vi "PolarizationSimulation.vi"() -> ()   [LabVIEW 2018]
uses:
  Sub-VI's/Adam_data.ctl
  <vilib>/Utility/xml.llb/Read From XML File(string).vi
  <vilib>/Utility/xml.llb/Write to XML File(string).vi
  <vilib>/Analysis/NI_AALBase.lvlib
panel:
  in  "Regularization":T1
  in  "Batch Size":i16
  out "NN Loss":dbl(graph)
  in  "Loss Function":enum16{"MSE", "MAE"}(ring)
  in  "Parameters File Path":path
  out "NN Error":dbl
  in  "Training?":bool
  out "NN Output":dbl
  in  "Speed\nMultiplier":dbl=1.0
  out "Rho_-":cluster{dbl[], "Array 3":dbl[]}(graph)
  out "Rho_0":cluster{dbl[], "Array out":dbl[]}(graph)
  in  "AFP On":bool
  in  "AFP Efficiency":dbl=0.9 min=0.0 max=1.0 step=0.01
  in  "AFP Control":cluster{i32, i32}(slide)={200, 230} scale=0.0..500.0
  out "lower R-value AFP":dbl
  out "upper R-value AFP":dbl
  in  "STOP":bool
  in  "Microwave Power":dbl=1.0
  in  "Lower Fit\nParameter":dbl=-3.6
  in  "Upper Fit\nParameter":dbl=3.6
  in  "Std Dev Noise":dbl step=0.0001
  out "lower R-value":dbl
  out "upper R-value":dbl
  in  "RF Control":cluster{i32, i32}(slide)={200, 230} scale=0.0..500.0
  out "p":dbl format="%_4g"
  out "r":dbl
  in  "Saturation\nPolarization":dbl=0.8 min=0.0 max=0.99 step=0.01
  out "Reimann \nsum of Q":dbl format="%_4g"
  out "Corrected Data (Q)":cluster{dbl[], dbl[]}(graph)
  out "Rho_+":cluster{dbl[], "Array out":dbl[]}(graph)
  in  "Select Target Type":u16(ring)=2 items=["Test Case", "Deuteron"]
  in  "Reset":bool
  out "Total Polarization (P)":cluster{dbl, dbl}(graph)
  in  "Spin Manipulation\nPower Factor":dbl=0.005
  in  "Decay Spin\nManipulation":bool
  out "Reimann\nsum of P":dbl format="%_4g"
  out "Corrected Data (P)":cluster{dbl[], dbl[]}[](graph)
  out "Signal and Fit (P)":cluster{dbl[], "Best Polynomial Fit":dbl[]}[](graph)
  in  "Positive\nPolarization":bool
  in  "Microwave on":bool
  # "Neural Network"
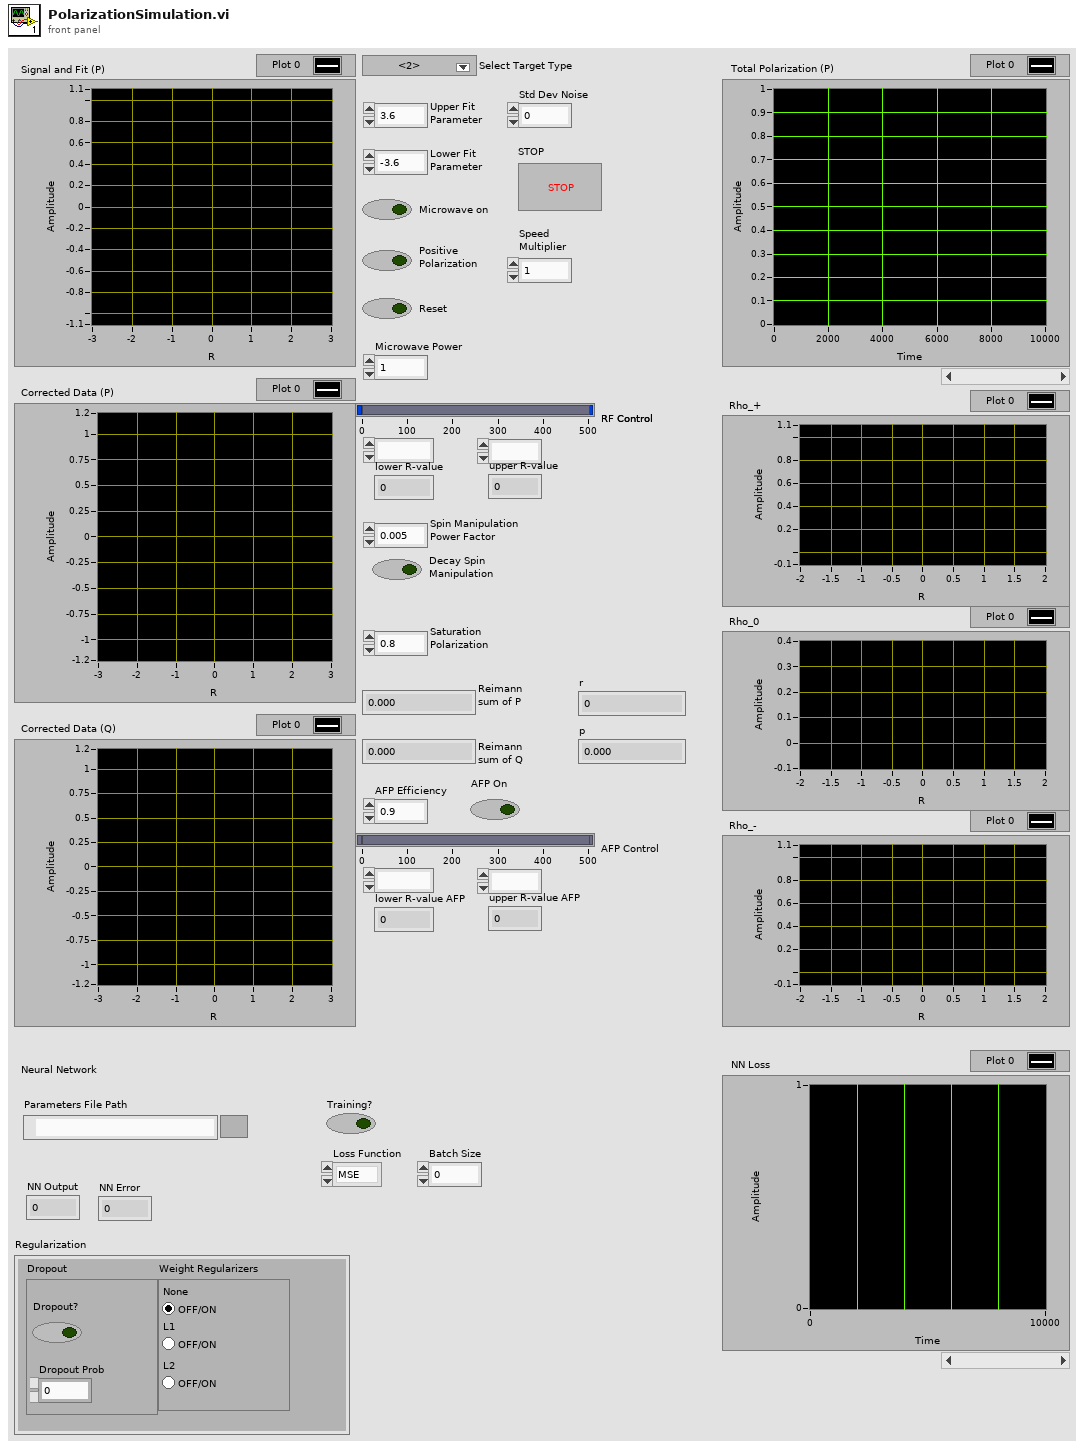
[diagram p1: front panel]
types:
  T1 = cluster{"Dropout":cluster{"Dropout?":bool, "Dropout Prob":dbl}, "Weight Regularizers":enum32{"None", "L1", "L2"}}
  T2 = typedef "Adam_data.ctl" = cluster{"Mw Moments":cluster{"3 ":dbl[], "2":dbl[][], "1":dbl[][]}, "Vw Moments":cluster{"3":dbl[], "2":dbl[][], "1":dbl[][]}, "Mb Moments":cluster{"3":dbl, "2":dbl[], "1":dbl[]}, "Vb Moments":cluster{"3":dbl, "2":dbl[], "1":dbl[]}}
  T3 = cluster{cluster{dbl[][], dbl[]}, cluster{dbl[][], dbl[]}, cluster{dbl[], dbl}}
  T4 = cluster{cluster{"Updated Weights":dbl[][], "Updated Biases":dbl[]}, cluster{"Updated Weights":dbl[][], "Updated Biases":dbl[]}, cluster{"Updated Weights":dbl[], "Updated Biases":dbl}}
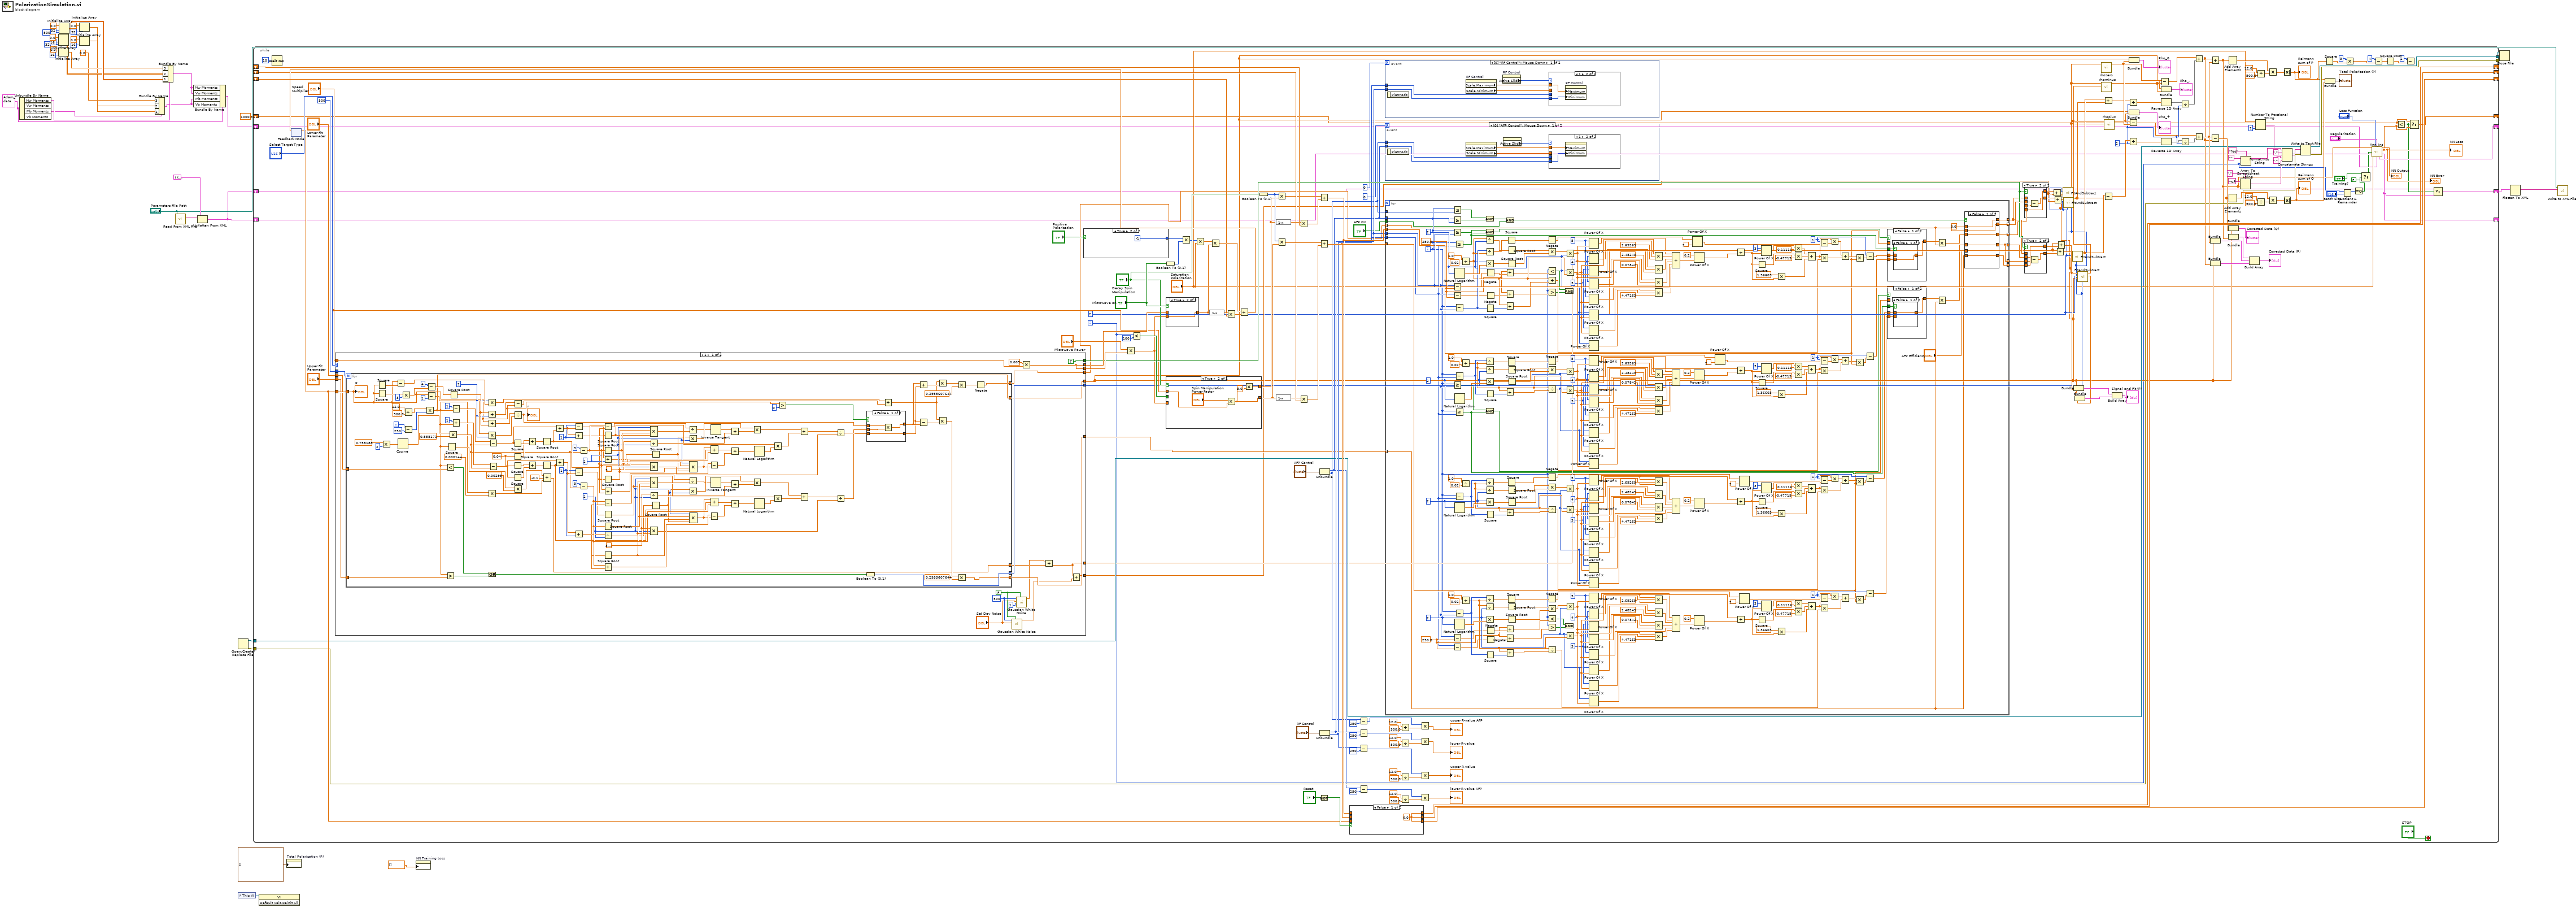
[diagram p0: block diagram]
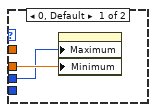
[diagram p2: hidden frame]
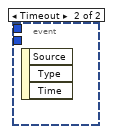
[diagram p3: hidden frame]
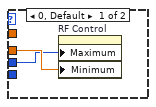
[diagram p4: hidden frame]
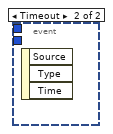
[diagram p5: hidden frame]
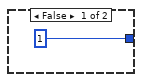
[diagram p6: hidden frame]
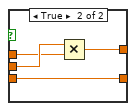
[diagram p7: hidden frame]
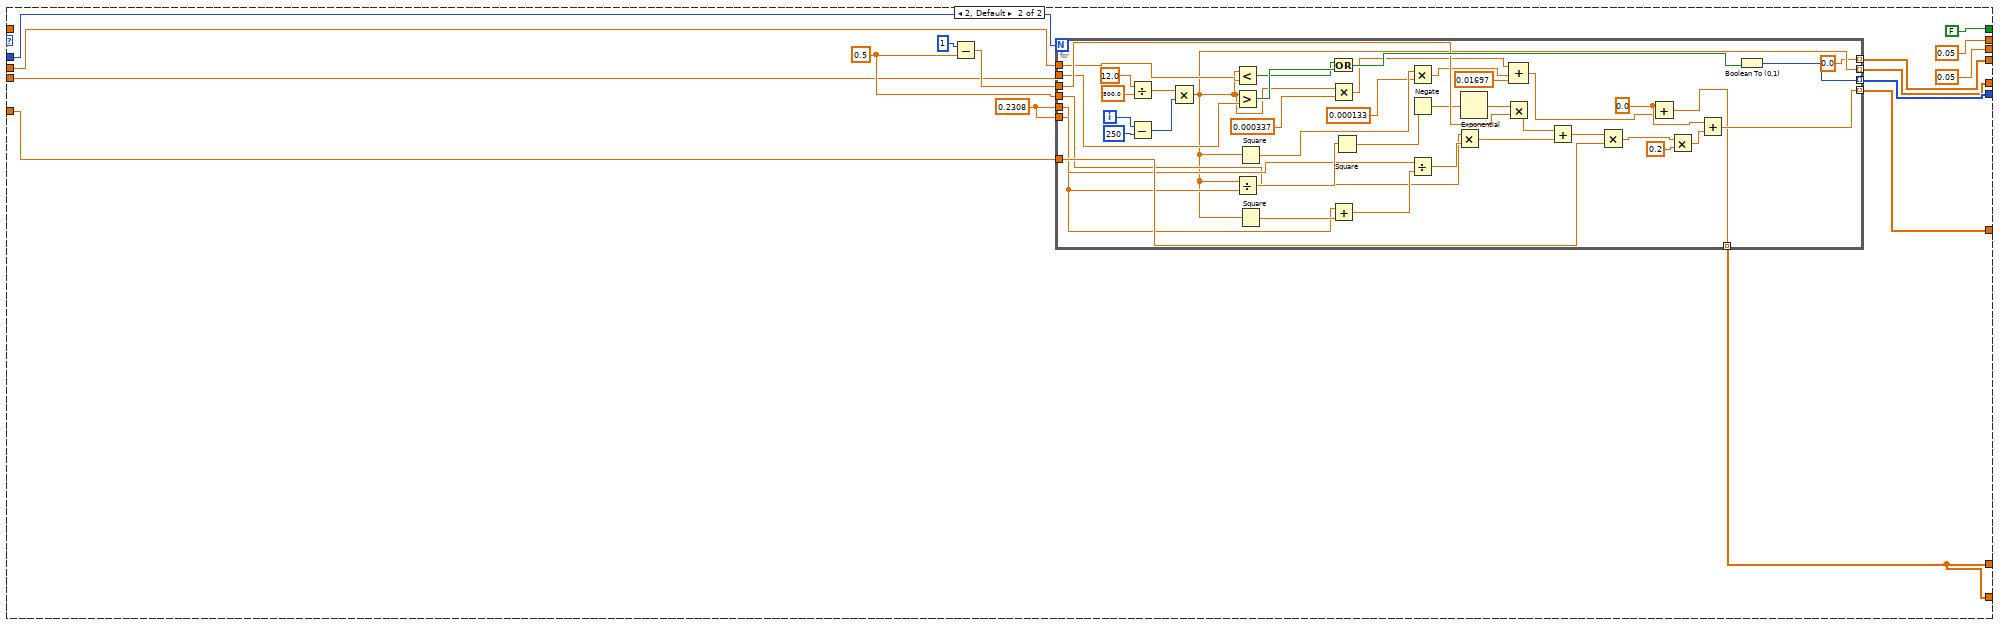
[diagram p8: hidden frame]
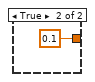
[diagram p10: hidden frame]
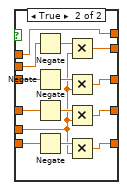
[diagram p15: hidden frame]
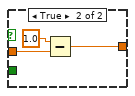
[diagram p17: hidden frame]
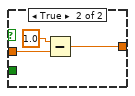
[diagram p19: hidden frame]
diagram:
  w7 = T2 {"Mw Moments"={"3 "=[], "2"=[], "1"=[]}, "Vw Moments"={"3"=[], "2"=[], "1"=[]}, "Mb Moments"={"3"=0.0, "2"=[], "1"=[]}, "Vb Moments"={"3"=0.0, "2"=[], "1"=[]}} ("Adam Data In")
  n1 = Unbundle By Name(w7) -> ("Mw Moments"=w9:cluster{"3 ":dbl[], "2":dbl[][], "1":dbl[][]}, "Mb Moments"=w8:cluster{"3":dbl, "2":dbl[], "1":dbl[]})  [unwired: 2 out]
  n2 = Initialize Array(0.0 ("element"), 16 ("dimension size"), 32 ("dimension size")) -> (w14:dbl[][])
  n3 = Initialize Array(0.0 ("element"), 16 ("dimension size")) -> (w13:dbl[])
  n4 = Initialize Array(0.0 ("element"), 32 ("dimension size"), 500 ("dimension size")) -> (w15:dbl[][])
  n5 = Initialize Array(0.0 ("element"), 16 ("dimension size")) -> (w11:dbl[])
  n6 = Initialize Array(0.0 ("element"), 32 ("dimension size")) -> (w12:dbl[])
  n7 = Bundle By Name(cluster=w8, "3"=0.0 ("element"), "2"=w11, "1"=w12) -> (w5:cluster{"3":dbl, "2":dbl[], "1":dbl[]})
  n8 = Bundle By Name(cluster=w9, "3"=w13, "2"=w14, "1"=w15) -> (w6:cluster{"3 ":dbl[], "2":dbl[][], "1":dbl[][]})
  n9 = call-poly <vilib>:"Read From XML File.vi"("XML File Path"="Parameters File Path") -> ("XML Elements"=w32:string)  [unwired: 8 in, 2 out]
  n10 = Bundle By Name(cluster=w7, "Mw Moments"=w6, "Vw Moments"=w6, "Mb Moments"=w5, "Vb Moments"=w5) -> (w4:T2)
  n11 = Unflatten From XML(xml string=w32, type=T3 {{[], []}, {[], []}, {[], 0.0}}) -> (value=w3:T3)  [unwired: 1 in, 1 out]
  n12 = Open/Create/Replace File() -> (refnum out=w36:refnum<file>, error out=w35:errorcluster)  [unwired: 6 in, 1 out]
  n13 = control-ref of="This VI"() -> (w38:refnum<vi>)
  n14 = while {
    shift-right: [w215] -> _
    shift-left: _ -> [w222]
    shift-right: [w214] -> _
    shift-left: _ -> [w197]
    shift-right: [w192] -> _
    shift-left: _ -> [w191]
    tunnel: w36 -> [w124]
    tunnel: w35 -> [w123]
    tunnel: [w122] -> w34
    tunnel: [w121] -> w33
    shift-right: [w42] -> _
    shift-left: w3 -> [w58]
    shift-right: [w55] -> _
    shift-left: w4 -> [w54]
    shift-right: [w46] -> _
    shift-left: 1000.0 ("Error") -> [w45]
    shift-right: [w41] -> w2
    shift-left: w3 -> [w40]
    i -> [w53]
    stop <- "STOP" stop-if-true
    w174 = 2
    w67 = 2
    n15 = Wait (ms)(milliseconds to wait=10) -> ()  [unwired: 1 out]
    n16 = feedback #1() -> (w201:dbl)  [unwired: 1 in]
    n17 = case shown="1" "Select Target Type" {
      tunnel: [w257 0.05 ("Growth Constant")] -> w206
      tunnel: [w257 0.05 ("Decay Constant")] -> w205
      tunnel: 500 -> [w266 w424]
      tunnel: w201 -> [w269 w423]
      tunnel: "Upper Fit\nParameter" -> [w267 w421]
      tunnel: "Lower Fit\nParameter" -> [w268 w422]
      tunnel: [w264 w419] -> w66
      tunnel: [w254 w418] -> w81
      tunnel: [w265 w420] -> w65
      tunnel: [TRUE FALSE] -> w185
      tunnel: [w255 w414] -> w80
      tunnel: "Speed\nMultiplier" -> [w256 _]
      tunnel: [w250 w413] -> w79
      tunnel: [w252 w413] -> w78
      frame 1 {
        w259 = FALSE
        w261 = 500
        n18 = for {
          N: w266 -> [_]
          tunnel: [w300] -> w264 mode=indexing
          tunnel: [w389] -> w265 mode=indexing
          tunnel: w267 -> [w388]
          tunnel: w268 -> [w387]
          tunnel: [w272] -> w254 mode=indexing
          tunnel: w269 -> [w273]
          tunnel: [w271] -> w255 mode=indexing
          tunnel: [w270] -> w253 mode=indexing
          i -> [w365]
          w287 = 2
          w326 = 1
          w330 = 3.141592653589793
          w324 = 2
          w309 = 0.04
          w362 = 1
          w367 = 3.141592653589793
          w360 = 2
          n19 = Square(x=w273) -> (x^2=w290:dbl)
          n20 = Square(x=w273) -> (x^2=w316:dbl)
          n21 = Multiply(x=0.758188, y=2) -> (x*y=w304:dbl)
          n22 = Subtract(x=w273, y=w290) -> (x-y=w289:dbl)
          n23 = Cosine(x=w304) -> (cos(x)=w307:dbl)
          n24 = Multiply(x=w316, y=3) -> (x*y=w315:dbl)
          n25 = Divide(x=12.0, y=500.0) -> (x/y=w403:dbl)
          n26 = Subtract(x=w365, y=250) -> (x-y=w402:i32)
          n27 = Multiply(x=w403, y=w402) -> (x*y=w300:dbl)
          n28 = Subtract(x=4, y=w315) -> (x-y=w313:dbl)
          n29 = Subtract(x=w273, y=1) -> (x-y=w311:dbl)
          n30 = Less?(x=w300, y=w387) -> (x < y?=w392:bool)
          n31 = Greater?(x=w300, y=w388) -> (0:w391:bool)
          n32 = Square(x=w300) -> (x^2=w302:dbl)
          n33 = Multiply(x=w307, y=0.558171) -> (x*y=w308:dbl)
          n34 = Square Root(x=w313) -> (sqrt(x)=w288:dbl)
          n35 = Subtract(x=1, y=w300) -> (x-y=w397:dbl)
          n36 = Add(x=1, y=w300) -> (x+y=w354:dbl)
          n37 = Multiply(x=w287, y=w289) -> (x*y=w285:dbl)
          n38 = Add(x=w288, y=w287) -> (x+y=w286:dbl)
          n39 = Add(x=w273, y=w288) -> (x+y=w312:dbl)
          n40 = Multiply(x=w311, y=w287) -> (x*y=w295:dbl)
          n41 = Multiply(x=w300, y=0.000144) -> (x*y=w297:dbl)
          n42 = Or(x=w392, y=w391) -> (x .or. y?=w390:bool)
          n43 = Subtract(x=w397, y=w308) -> (x-y=w393:dbl)
          n44 = Subtract(x=w354, y=w308) -> (x-y=w350:dbl)
          n45 = Square(x=w393) -> (x^2=w396:dbl)
          n46 = Square(x=w309) -> (x^2=w395:dbl)
          n47 = Square(x=w309) -> (x^2=w352:dbl)
          n48 = Square(x=w350) -> (x^2=w353:dbl)
          n49 = Subtract(x=w286, y=w273) -> (x-y=w284:dbl)
          n50 = Divide(x=w312, y=w295) -> (x/y=w291:dbl)
          "r" <- w291
          n51 = Multiply(x=w302, y=0.00295) -> (x*y=w301:dbl)
          n52 = Add(x=w395, y=w396) -> (x+y=w394:dbl)
          n53 = Add(x=w352, y=w353) -> (x+y=w351:dbl)
          n54 = Square Root(x=w394) -> (sqrt(x)=w357:dbl)
          n55 = Square Root(x=w351) -> (sqrt(x)=w321:dbl)
          n56 = Compound Arithmetic op=ADD(w301, -0.1, w297) -> (w270:dbl)
          n57 = Divide(x=w393, y=w357) -> (x/y=w363:dbl)
          n58 = Divide(x=w350, y=w321) -> (x/y=w327:dbl)
          n59 = Subtract(x=w362, y=w363) -> (x-y=w318:dbl)
          n60 = Add(x=w363, y=w362) -> (x+y=w361:dbl)
          n61 = Subtract(x=w326, y=w327) -> (x-y=w319:dbl)
          n62 = Add(x=w327, y=w326) -> (x+y=w325:dbl)
          n63 = Subtract(x=3, y=w308) -> (x-y=w373:dbl)
          n64 = Subtract(x=3, y=w308) -> (x-y=w336:dbl)
          n65 = Subtract(x=w373, y=w357) -> (x-y=w382:dbl)
          n66 = Square Root(x=w318) -> (sqrt(x)=w364:dbl)
          n67 = Square Root(x=w373) -> (sqrt(x)=w376:dbl)
          n68 = Divide(x=w361, y=w360) -> (x/y=w359:dbl)
          n69 = Square Root(x=w357) -> (sqrt(x)=w366:dbl)
          n70 = Add(x=w373, y=w357) -> (x+y=w372:dbl)
          n71 = Subtract(x=w336, y=w321) -> (x-y=w345:dbl)
          n72 = Square Root(x=w319) -> (sqrt(x)=w328:dbl)
          n73 = Square Root(x=w336) -> (sqrt(x)=w339:dbl)
          n74 = Divide(x=w325, y=w324) -> (x/y=w323:dbl)
          n75 = Square Root(x=w321) -> (sqrt(x)=w329:dbl)
          n76 = Add(x=w336, y=w321) -> (x+y=w335:dbl)
          n77 = Divide(x=w367, y=w360) -> (x/y=w384:dbl)
          n78 = Divide(x=w330, y=w324) -> (x/y=w347:dbl)
          n79 = Compound Arithmetic op=MULTIPLY(w360, w366, w376, w364) -> (w381:dbl)
          n80 = Compound Arithmetic op=MULTIPLY(w367, w360, w366) -> (w368:dbl)
          n81 = Compound Arithmetic op=MULTIPLY(w324, w329, w339, w328) -> (w344:dbl)
          n82 = Compound Arithmetic op=MULTIPLY(w330, w324, w329) -> (w331:dbl)
          n83 = Square Root(x=w359) -> (sqrt(x)=w358:dbl)
          n84 = Square Root(x=w323) -> (sqrt(x)=w322:dbl)
          n85 = Divide(x=w382, y=w381) -> (x/y=w380:dbl)
          n86 = Multiply(x=w358, y=w360) -> (x*y=w386:dbl)
          n87 = Divide(x=w345, y=w344) -> (x/y=w343:dbl)
          n88 = Multiply(x=w322, y=w324) -> (x*y=w349:dbl)
          n89 = Compound Arithmetic op=MULTIPLY(w360, w376, w366, w358) -> (w371:dbl)
          n90 = Compound Arithmetic op=MULTIPLY(w324, w339, w329, w322) -> (w334:dbl)
          n91 = Subtract(x=w372, y=w371) -> (x-y=w370:dbl)
          n92 = Subtract(x=w335, y=w334) -> (x-y=w333:dbl)
          n93 = Inverse Tangent(1:w380) -> (0:w385:dbl)
          n94 = Compound Arithmetic op=ADD(w371, w357, w373) -> (w375:dbl)
          n95 = Inverse Tangent(1:w343) -> (0:w348:dbl)
          n96 = Compound Arithmetic op=ADD(w334, w321, w336) -> (w338:dbl)
          n97 = Add(x=w385, y=w384) -> (x+y=w383:dbl)
          n98 = Divide(x=w375, y=w370) -> (x/y=w374:dbl)
          n99 = Add(x=w348, y=w347) -> (x+y=w346:dbl)
          n100 = Divide(x=w338, y=w333) -> (x/y=w337:dbl)
          n101 = Multiply(x=w386, y=w383) -> (x*y=w379:dbl)
          n102 = Multiply(x=w349, y=w346) -> (x*y=w342:dbl)
          n103 = Natural Logarithm(1:w374) -> (0:w377:dbl)
          n104 = Natural Logarithm(1:w337) -> (0:w340:dbl)
          n105 = Multiply(x=w364, y=w377) -> (x*y=w378:dbl)
          n106 = Multiply(x=w328, y=w340) -> (x*y=w341:dbl)
          n107 = Greater?(x=w273, y=0) -> (0:w275:bool)
          n108 = Add(x=w379, y=w378) -> (x+y=w369:dbl)
          n109 = Add(x=w342, y=w341) -> (x+y=w332:dbl)
          n110 = Divide(x=w369, y=w368) -> (x/y=w310:dbl)
          n111 = Divide(x=w332, y=w331) -> (x/y=w277:dbl)
          n112 = Boolean To (0,1)(Boolean=w390) -> (0, 1=w389:i16)
          n113 = case shown="False" w275 {
            tunnel: w310 -> [w407 w412]
            tunnel: [w405 w411] -> w293
            tunnel: w291 -> [w408 w410]
            tunnel: w277 -> [w406 w409]
            tunnel: [w406 w409] -> w276
            frame False {
              n114 = Multiply(x=w408, y=w407) -> (x*y=w405:dbl)
            }
            frame True {
              n115 = Multiply(x=w412, y=w410) -> (x*y=w411:dbl)
            }
          }
          n116 = Divide(x=w285, y=w284) -> (x/y=w283:dbl)
          n117 = Add(x=w293, y=w276) -> (x+y=w294:dbl)
          n118 = Subtract(x=w276, y=w293) -> (x-y=w320:dbl)
          n119 = Multiply(x=w283, y=w294) -> (x*y=w282:dbl)
          n120 = Multiply(x=w283, y=w320) -> (x*y=w281:dbl)
          n121 = Multiply(x=w282, y=0.2955607644) -> (x*y=w280:dbl)
          n122 = Multiply(x=w281, y=0.2955607644) -> (x*y=w272:dbl)
          n123 = Negate(x=w280) -> (-x=w271:dbl)
          "p" <- w273
        }
        n124 = call <vilib>:"Gaussian White Noise.vi"("initialize?"=w259, "standard deviation"="Std Dev Noise", "samples"=w261) -> ("Gaussian noise pattern"=w251:dbl[])  [unwired: 7 in, 1 out]
        n125 = call <vilib>:"Gaussian White Noise.vi"("initialize?"=w259, "seed"=1, "standard deviation"="Std Dev Noise", "samples"=w261) -> ("Gaussian noise pattern"=w249:dbl[])  [unwired: 6 in, 1 out]
        n126 = Multiply(x=0.005, y=w256) -> (x*y=w257:dbl)
        n127 = Add(x=w249, y=w253) -> (x+y=w250:dbl[])
        n128 = Add(x=w250, y=w251) -> (x+y=w252:dbl[])
      }
      frame 2, Default {
        w425 = 0.2308
        w426 = 0.5
        n129 = Subtract(x=1, y=w426) -> (x-y=w428:dbl)
        n130 = for {
          N: w424 -> [_]
          tunnel: w423 -> [w468]
          tunnel: [w434] -> w419 mode=indexing
          tunnel: [w452] -> w418 mode=indexing
          tunnel: [w466] -> w420 mode=indexing
          tunnel: w428 -> [w462]
          tunnel: w425 -> [w460]
          tunnel: w425 -> [w441]
          tunnel: w426 -> [w454]
          tunnel: w421 -> [w449]
          tunnel: w422 -> [w448]
          tunnel: [0.0] -> w414 mode=indexing
          tunnel: [w429] -> w413 mode=indexing
          i -> [w442]
          w453 = 0.0
          n131 = Divide(x=12.0, y=500.0) -> (x/y=w443:dbl)
          n132 = Subtract(x=w442, y=250) -> (x-y=w447:i32)
          n133 = Multiply(x=w443, y=w447) -> (x*y=w434:dbl)
          n134 = Less?(x=w434, y=w448) -> (x < y?=w463:bool)
          n135 = Greater?(x=w434, y=w449) -> (0:w464:bool)
          n136 = Divide(x=w434, y=w441) -> (x/y=w469:dbl)
          n137 = Square(x=w434) -> (x^2=w437:dbl)
          n138 = Square(x=w434) -> (x^2=w459:dbl)
          n139 = Or(x=w463, y=w464) -> (x .or. y?=w465:bool)
          n140 = Multiply(x=w434, y=0.000337) -> (x*y=w436:dbl)
          n141 = Add(x=w441, y=w459) -> (x+y=w461:dbl)
          n142 = Square(x=w469) -> (x^2=w470:dbl)
          n143 = Multiply(x=w437, y=0.000133) -> (x*y=w435:dbl)
          n144 = Negate(x=w470) -> (-x=w451:dbl)
          n145 = Divide(x=w460, y=w461) -> (x/y=w456:dbl)
          n146 = Multiply(x=w454, y=w456) -> (x*y=w455:dbl)
          n147 = Exponential(1:w451) -> (0:w450:dbl)
          n148 = Multiply(x=w450, y=w462) -> (x*y=w458:dbl)
          n149 = Compound Arithmetic op=ADD(w436, w435, 0.01697) -> (w438:dbl)
          n150 = Add(x=w458, y=w455) -> (x+y=w457:dbl)
          n151 = Multiply(x=w457, y=w468) -> (x*y=w467:dbl)
          n152 = Add(x=w453, y=w438) -> (x+y=w429:dbl)
          n153 = Multiply(x=w467, y=0.2) -> (x*y=w440:dbl)
          n154 = Add(x=w453, y=w440) -> (x+y=w452:dbl)
          n155 = Boolean To (0,1)(Boolean=w465) -> (0, 1=w466:i16)
        }
      }
    }
    n156 = case shown="True" "Positive\nPolarization" {
      tunnel: [1 -1] -> w159
      frame False {
      }
      frame True {
      }
    }
    n157 = Multiply(x="Microwave Power", y=w206) -> (x*y=w127:dbl)
    n158 = Less?(x=w53, y=100) -> (x < y?=w217:bool)
    n159 = Boolean To (0,1)(Boolean="Microwave on") -> (0, 1=w224:i16)
    n160 = case shown="True" "Microwave on" {
      tunnel: [w481 w482] -> w209
      tunnel: w127 -> [_ w482]
      tunnel: w205 -> [w481 _]
      frame False {
      }
      frame True {
      }
    }
    n161 = case shown="True" "Decay Spin\nManipulation" {
      tunnel: [w471 w477] -> w218
      tunnel: w127 -> [w473 _]
      tunnel: w217 -> [w472 _]
      tunnel: [w471 w478] -> w199
      tunnel: "Speed\nMultiplier" -> [_ w476]
      frame False {
        n162 = case shown="False" w472 {
          tunnel: [w474 0.1] -> w471
          tunnel: w473 -> [w474 _]
          frame False {
          }
          frame True {
          }
        }
      }
      frame True {
        n163 = Multiply(x="Spin Manipulation\nPower Factor", y=w476) -> (x*y=w477:dbl)
        n164 = Multiply(x=w477, y=3.0) -> (x*y=w478:dbl)
      }
    }
    n165 = Multiply(x=w159, y=w224) -> (x*y=w160:i32)
    n166 = Multiply(x=w160, y="Saturation\nPolarization") -> (x*y=w167:dbl)
    n167 = expression code="1-x"(w209) -> (w225:dbl)
    n168 = Multiply(x=w167, y=w209) -> (x*y=w226:dbl)
    n169 = Multiply(x=w225, y=w222) -> (x*y=w227:dbl)
    n170 = Add(x=w226, y=w227) -> (x+y=w204:dbl)
    n171 = feedback-in #1(w204) -> ()
    n172 = Boolean To (0,1)(Boolean="Decay Spin\nManipulation") -> (0, 1=w200:i16)
    n173 = expression code="1-x"(w199) -> (w198:dbl)
    n174 = expression code="1-x"(w218) -> (w219:dbl)
    n175 = Multiply(x=w200, y=w199) -> (x*y=w195:dbl)
    n176 = Multiply(x=w200, y=w218) -> (x*y=w220:dbl)
    n177 = Multiply(x=w198, y=w191) -> (x*y=w196:dbl)
    n178 = Multiply(x=w219, y=w197) -> (x*y=w221:dbl)
    n179 = Add(x=w195, y=w196) -> (x+y=w193:dbl)
    n180 = Add(x=w220, y=w221) -> (x+y=w213:dbl)
    n181 = Not(x="Reset") -> (.not. x?=w212:bool)
    n182 = Unbundle("AFP Control") -> (w91:i32, w90:i32)
    n183 = Unbundle("RF Control") -> (w130:i32, w129:i32)
    n184 = case shown="False" w212 {
      tunnel: [w495 w498] -> w215
      tunnel: w201 -> [_ w498]
      tunnel: [w495 w497] -> w214
      tunnel: w213 -> [_ w497]
      tunnel: w193 -> [_ w496]
      tunnel: [w495 w496] -> w192
      frame False {
        w495 = 0.0
      }
      frame True {
      }
    }
    n185 = Subtract(x=w90, y=250) -> (x-y=w97:i32)
    n186 = Subtract(x=w130, y=250) -> (x-y=w136:i32)
    n187 = Subtract(x=w129, y=250) -> (x-y=w139:i32)
    n188 = Subtract(x=w91, y=250) -> (x-y=w94:i32)
    n189 = event shown="[0] \"RF Control\": Mouse Down" {
      selector: _ -> [_ _]
      dyn-events: _ -> [_ _]
      timeout: 0 -> [_ _]
      tunnel: w130 -> [w239 _]
      tunnel: w129 -> [w238 _]
      event "RF Control": Mouse Down {
        n190 = event-data() -> ()  [unwired: 1 in, 1 out]
        n191 = property on="RF Control" class="Slide (strict)"() -> ("Scale.Maximum"=w240:dbl, "Scale.Minimum"=w241:dbl)  [unwired: 2 in, 2 out]
        n192 = property on="RF Control" class="Slide (strict)"() -> ("Active Slider"=w242:i32)  [unwired: 2 in, 2 out]
        n193 = case shown="1" w242 {
          tunnel: w241 -> [w244 _]
          tunnel: w238 -> [w243 _]
          tunnel: w240 -> [_ w246]
          tunnel: w239 -> [_ w245]
          frame 0, Default {
            n194 = property on="RF Control" class="Slide (strict)"("Maximum"=w243, "Minimum"=w244) -> ()  [unwired: 2 in, 2 out]
          }
          frame 1 {
            n195 = property on="RF Control" class="Slide (strict)"("Maximum"=w246, "Minimum"=w245) -> ()  [unwired: 2 in, 2 out]
          }
        }
      }
      event Timeout {
        n196 = event-data() -> ()  [unwired: 1 in, 3 out]
      }
    }
    n197 = event shown="[0] \"AFP Control\": Mouse Down" {
      selector: _ -> [_ _]
      dyn-events: _ -> [_ _]
      timeout: 0 -> [_ _]
      tunnel: w91 -> [w230 _]
      tunnel: w90 -> [w229 _]
      event "AFP Control": Mouse Down {
        n198 = event-data() -> ()  [unwired: 1 in, 1 out]
        n199 = property on="AFP Control" class="Slide (strict)"() -> ("Scale.Maximum"=w231:dbl, "Scale.Minimum"=w232:dbl)  [unwired: 2 in, 2 out]
        n200 = property on="AFP Control" class="Slide (strict)"() -> ("Active Slider"=w233:i32)  [unwired: 2 in, 2 out]
        n201 = case shown="1" w233 {
          tunnel: w232 -> [w235 _]
          tunnel: w229 -> [w234 _]
          tunnel: w231 -> [_ w237]
          tunnel: w230 -> [_ w236]
          frame 0, Default {
            n202 = property on="AFP Control" class="Slide (strict)"("Maximum"=w234, "Minimum"=w235) -> ()  [unwired: 2 in, 2 out]
          }
          frame 1 {
            n203 = property on="AFP Control" class="Slide (strict)"("Maximum"=w237, "Minimum"=w236) -> ()  [unwired: 2 in, 2 out]
          }
        }
      }
      event Timeout {
        n204 = event-data() -> ()  [unwired: 1 in, 3 out]
      }
    }
    n205 = for {
      tunnel: w81 -> [w511] mode=indexing
      tunnel: w213 -> [w663]
      tunnel: w129 -> [w521]
      tunnel: w130 -> [w520]
      tunnel: [w507] -> w203 mode=indexing
      tunnel: [w508] -> w194 mode=indexing
      tunnel: [w508] -> w202 mode=indexing
      tunnel: w80 -> [w500] mode=indexing
      tunnel: w193 -> [w519]
      tunnel: [w499] -> w189 mode=indexing
      tunnel: [w506] -> w179 mode=indexing
      tunnel: w91 -> [w515]
      tunnel: w90 -> [w514]
      tunnel: "AFP On" -> [w503]
      tunnel: [w502] -> w88 mode=indexing
      i -> [w513]
      w523 = 250.0
      w562 = 5
      w560 = 4
      w559 = 3
      w540 = 1
      w541 = 2
      w623 = 5
      w621 = 4
      w620 = 3
      w600 = 1
      w601 = 2
      w657 = 250.0
      w698 = 5
      w696 = 4
      w695 = 3
      w676 = 1
      w677 = 2
      w759 = 5
      w757 = 4
      w756 = 3
      w736 = 1
      w737 = 2
      n206 = Less Or Equal?(x=w513, y=w514) -> (x <= y?=w516:bool)
      n207 = Greater Or Equal?(x=w513, y=w515) -> (x >= y?=w517:bool)
      n208 = Greater Or Equal?(x=w513, y=w520) -> (x >= y?=w596:bool)
      n209 = Subtract(x=w520, y=w523) -> (x-y=w527:dbl)
      n210 = Subtract(x=w521, y=w523) -> (x-y=w528:dbl)
      n211 = Greater Or Equal?(x=w513, y=w520) -> (x >= y?=w732:bool)
      n212 = Subtract(x=w520, y=w657) -> (x-y=w661:dbl)
      n213 = Subtract(x=w521, y=w657) -> (x-y=w662:dbl)
      n214 = Less Or Equal?(x=w513, y=w521) -> (x <= y?=w533:bool)
      n215 = Natural Logarithm(1:w601) -> (0:w636:dbl)
      n216 = Subtract(x=w513, y=w520) -> (x-y=w609:i32)
      n217 = Subtract(x=w513, y=w521) -> (x-y=w548:i32)
      n218 = Natural Logarithm(1:w541) -> (0:w575:dbl)
      n219 = Less Or Equal?(x=w513, y=w521) -> (x <= y?=w668:bool)
      n220 = Subtract(x=w513, y=w521) -> (x-y=w684:i32)
      n221 = Natural Logarithm(1:w677) -> (0:w711:dbl)
      n222 = Subtract(x=w513, y=w520) -> (x-y=w745:i32)
      n223 = Natural Logarithm(1:w737) -> (0:w772:dbl)
      n224 = Divide(x=1.0, y=0.02) -> (x/y=w605:dbl)
      n225 = Divide(x=1.0, y=0.02) -> (x/y=w545:dbl)
      n226 = Divide(x=1.0, y=0.02) -> (x/y=w681:dbl)
      n227 = Divide(x=1.0, y=0.02) -> (x/y=w741:dbl)
      n228 = And(x=w516, y=w517) -> (x .and. y?=w505:bool)
      n229 = And(x=w596, y=w533) -> (x .and. y?=w534:bool)
      n230 = Divide(x=w605, y=w601) -> (x/y=w634:dbl)
      n231 = Divide(x=w609, y=w605) -> (x/y=w613:dbl)
      n232 = Multiply(x=w601, y=w636) -> (x*y=w637:dbl)
      n233 = Divide(x=w548, y=w545) -> (x/y=w552:dbl)
      n234 = Divide(x=w545, y=w541) -> (x/y=w573:dbl)
      n235 = Multiply(x=w541, y=w575) -> (x*y=w576:dbl)
      n236 = And(x=w732, y=w668) -> (x .and. y?=w670:bool)
      n237 = Divide(x=w684, y=w681) -> (x/y=w688:dbl)
      n238 = Divide(x=w681, y=w677) -> (x/y=w709:dbl)
      n239 = Multiply(x=w677, y=w711) -> (x*y=w712:dbl)
      n240 = Divide(x=w745, y=w741) -> (x/y=w749:dbl)
      n241 = Divide(x=w741, y=w737) -> (x/y=w770:dbl)
      n242 = Multiply(x=w737, y=w772) -> (x*y=w773:dbl)
      n243 = Square(x=w609) -> (x^2=w610:i32)
      n244 = Square(x=w548) -> (x^2=w549:i32)
      n245 = Square(x=w684) -> (x^2=w685:i32)
      n246 = Square(x=w745) -> (x^2=w746:i32)
      n247 = Negate(x=w527) -> (-x=w526:dbl)
      n248 = Negate(x=w528) -> (-x=w524:dbl)
      n249 = Negate(x=w661) -> (-x=w660:dbl)
      n250 = Negate(x=w662) -> (-x=w658:dbl)
      n251 = Add(x=w523, y=w526) -> (x+y=w525:dbl)
      n252 = Add(x=w523, y=w524) -> (x+y=w522:dbl)
      n253 = Add(x=w605, y=w610) -> (x+y=w611:dbl)
      n254 = Add(x=w545, y=w549) -> (x+y=w550:dbl)
      n255 = Add(x=w681, y=w685) -> (x+y=w686:dbl)
      n256 = Add(x=w657, y=w660) -> (x+y=w659:dbl)
      n257 = Add(x=w657, y=w658) -> (x+y=w656:dbl)
      n258 = Add(x=w741, y=w746) -> (x+y=w747:dbl)
      n259 = And(x=w505, y=w503) -> (x .and. y?=w504:bool)
      n260 = Square(x=w613) -> (x^2=w615:dbl)
      n261 = Square(x=w552) -> (x^2=w554:dbl)
      n262 = Square(x=w688) -> (x^2=w690:dbl)
      n263 = Square(x=w749) -> (x^2=w751:dbl)
      n264 = Square Root(x=w634) -> (sqrt(x)=w635:dbl)
      n265 = Square Root(x=w637) -> (sqrt(x)=w638:dbl)
      n266 = Square Root(x=w573) -> (sqrt(x)=w574:dbl)
      n267 = Square Root(x=w576) -> (sqrt(x)=w577:dbl)
      n268 = Square Root(x=w709) -> (sqrt(x)=w710:dbl)
      n269 = Square Root(x=w712) -> (sqrt(x)=w713:dbl)
      n270 = Square Root(x=w770) -> (sqrt(x)=w771:dbl)
      n271 = Square Root(x=w773) -> (sqrt(x)=w774:dbl)
      n272 = Negate(x=w615) -> (-x=w614:dbl)
      n273 = Multiply(x=w635, y=w638) -> (x*y=w629:dbl)
      n274 = Less?(x=w513, y=w525) -> (x < y?=w530:bool)
      n275 = Divide(x=w605, y=w611) -> (x/y=w608:dbl)
      n276 = Greater?(x=w513, y=w522) -> (0:w529:bool)
      n277 = Negate(x=w554) -> (-x=w553:dbl)
      n278 = Multiply(x=w574, y=w577) -> (x*y=w568:dbl)
      n279 = Divide(x=w545, y=w550) -> (x/y=w535:dbl)
      n280 = Negate(x=w690) -> (-x=w689:dbl)
      n281 = Multiply(x=w710, y=w713) -> (x*y=w704:dbl)
      n282 = Divide(x=w681, y=w686) -> (x/y=w671:dbl)
      n283 = Negate(x=w751) -> (-x=w750:dbl)
      n284 = Multiply(x=w771, y=w774) -> (x*y=w765:dbl)
      n285 = Less?(x=w513, y=w659) -> (x < y?=w665:bool)
      n286 = Greater?(x=w513, y=w656) -> (0:w664:bool)
      n287 = Divide(x=w741, y=w747) -> (x/y=w744:dbl)
      n288 = And(x=w530, y=w529) -> ()  [unwired: 1 out]
      n289 = And(x=w665, y=w664) -> ()  [unwired: 1 out]
      n290 = Multiply(x=w629, y=w601) -> (x*y=w653:dbl)
      n291 = Multiply(x=w601, y=w605) -> (x*y=w647:dbl)
      n292 = Multiply(x=w568, y=w541) -> (x*y=w592:dbl)
      n293 = Multiply(x=w541, y=w545) -> (x*y=w586:dbl)
      n294 = Multiply(x=w704, y=w677) -> (x*y=w728:dbl)
      n295 = Multiply(x=w677, y=w681) -> (x*y=w722:dbl)
      n296 = Multiply(x=w765, y=w737) -> (x*y=w789:dbl)
      n297 = Multiply(x=w737, y=w741) -> (x*y=w783:dbl)
      n298 = Power Of X(1:w653, 2:w623) -> (0:w640:dbl)
      n299 = Power Of X(1:w653, 2:w621) -> (0:w646:dbl)
      n300 = Power Of X(1:w653, 2:w620) -> (0:w648:dbl)
      n301 = Power Of X(1:w647, 2:w621) -> (0:w652:dbl)
      n302 = Power Of X(1:w647, 2:w623) -> (0:w641:dbl)
      n303 = Power Of X(1:w647, 2:w601) -> (0:w649:dbl)
      n304 = Power Of X(1:w647, 2:w620) -> (0:w650:dbl)
      n305 = Power Of X(1:w653, 2:w601) -> (0:w651:dbl)
      n306 = Power Of X(1:w592, 2:w562) -> (0:w579:dbl)
      n307 = Power Of X(1:w592, 2:w560) -> (0:w585:dbl)
      n308 = Power Of X(1:w592, 2:w559) -> (0:w587:dbl)
      n309 = Power Of X(1:w586, 2:w560) -> (0:w591:dbl)
      n310 = Power Of X(1:w586, 2:w562) -> (0:w580:dbl)
      n311 = Power Of X(1:w586, 2:w541) -> (0:w588:dbl)
      n312 = Power Of X(1:w586, 2:w559) -> (0:w589:dbl)
      n313 = Power Of X(1:w592, 2:w541) -> (0:w590:dbl)
      n314 = Power Of X(1:w728, 2:w698) -> (0:w715:dbl)
      n315 = Power Of X(1:w728, 2:w696) -> (0:w721:dbl)
      n316 = Power Of X(1:w728, 2:w695) -> (0:w723:dbl)
      n317 = Power Of X(1:w722, 2:w696) -> (0:w727:dbl)
      n318 = Power Of X(1:w722, 2:w698) -> (0:w716:dbl)
      n319 = Power Of X(1:w722, 2:w677) -> (0:w724:dbl)
      n320 = Power Of X(1:w722, 2:w695) -> (0:w725:dbl)
      n321 = Power Of X(1:w728, 2:w677) -> (0:w726:dbl)
      n322 = Power Of X(1:w789, 2:w759) -> (0:w776:dbl)
      n323 = Power Of X(1:w789, 2:w757) -> (0:w782:dbl)
      n324 = Power Of X(1:w789, 2:w756) -> (0:w784:dbl)
      n325 = Power Of X(1:w783, 2:w757) -> (0:w788:dbl)
      n326 = Power Of X(1:w783, 2:w759) -> (0:w777:dbl)
      n327 = Power Of X(1:w783, 2:w737) -> (0:w785:dbl)
      n328 = Power Of X(1:w783, 2:w756) -> (0:w786:dbl)
      n329 = Power Of X(1:w789, 2:w737) -> (0:w787:dbl)
      n330 = Compound Arithmetic op=MULTIPLY(w647, w646, 2.69269) -> (w642:dbl)
      n331 = Compound Arithmetic op=MULTIPLY(w648, w649, 2.48243) -> (w644:dbl)
      n332 = Compound Arithmetic op=MULTIPLY(w653, w652, 0.07842) -> (w643:dbl)
      n333 = Compound Arithmetic op=MULTIPLY(w650, w651, 4.47163) -> (w645:dbl)
      n334 = Compound Arithmetic op=MULTIPLY(w586, w585, 2.69269) -> (w581:dbl)
      n335 = Compound Arithmetic op=MULTIPLY(w587, w588, 2.48243) -> (w583:dbl)
      n336 = Compound Arithmetic op=MULTIPLY(w592, w591, 0.07842) -> (w582:dbl)
      n337 = Compound Arithmetic op=MULTIPLY(w589, w590, 4.47163) -> (w584:dbl)
      n338 = Compound Arithmetic op=MULTIPLY(w722, w721, 2.69269) -> (w717:dbl)
      n339 = Compound Arithmetic op=MULTIPLY(w723, w724, 2.48243) -> (w719:dbl)
      n340 = Compound Arithmetic op=MULTIPLY(w728, w727, 0.07842) -> (w718:dbl)
      n341 = Compound Arithmetic op=MULTIPLY(w725, w726, 4.47163) -> (w720:dbl)
      n342 = Compound Arithmetic op=MULTIPLY(w783, w782, 2.69269) -> (w778:dbl)
      n343 = Compound Arithmetic op=MULTIPLY(w784, w785, 2.48243) -> (w780:dbl)
      n344 = Compound Arithmetic op=MULTIPLY(w789, w788, 0.07842) -> (w779:dbl)
      n345 = Compound Arithmetic op=MULTIPLY(w786, w787, 4.47163) -> (w781:dbl)
      n346 = Compound Arithmetic op=unknown(w640, w642, w644, w643, w641, w645) -> (w602:dbl)
      n347 = Compound Arithmetic op=unknown(w579, w581, w583, w582, w580, w584) -> (w542:dbl)
      n348 = Compound Arithmetic op=unknown(w715, w717, w719, w718, w716, w720) -> (w678:dbl)
      n349 = Compound Arithmetic op=unknown(w776, w778, w780, w779, w777, w781) -> (w738:dbl)
      n350 = Power Of X(1:2.718281828459045, 2:w614) -> (0:w612:dbl)
      n351 = Power Of X(1:w602, 2:0.2) -> (0:w655:dbl)
      n352 = Power Of X(1:w542, 2:0.2) -> (0:w594:dbl)
      n353 = Power Of X(1:w678, 2:0.2) -> (0:w730:dbl)
      n354 = Power Of X(1:w738, 2:0.2) -> (0:w791:dbl)
      n355 = Power Of X(1:2.718281828459045, 2:w553) -> (0:w551:dbl)
      n356 = Divide(x=w647, y=w655) -> (x/y=w639:dbl)
      n357 = Divide(x=w586, y=w594) -> (x/y=w578:dbl)
      n358 = Divide(x=w722, y=w730) -> (x/y=w714:dbl)
      n359 = Divide(x=w783, y=w791) -> (x/y=w775:dbl)
      n360 = Power Of X(1:2.718281828459045, 2:w689) -> (0:w687:dbl)
      n361 = Power Of X(1:2.718281828459045, 2:w750) -> (0:w748:dbl)
      n362 = Square(x=w639) -> (x^2=w633:dbl)
      n363 = Square(x=w578) -> (x^2=w572:dbl)
      n364 = Square(x=w714) -> (x^2=w708:dbl)
      n365 = Square(x=w775) -> (x^2=w769:dbl)
      n366 = Power Of X(1:w639, 2:3) -> (0:w632:dbl)
      n367 = Power Of X(1:w578, 2:3) -> (0:w571:dbl)
      n368 = Power Of X(1:w714, 2:3) -> (0:w707:dbl)
      n369 = Power Of X(1:w775, 2:3) -> (0:w768:dbl)
      n370 = Multiply(x=1.36603, y=w639) -> (x*y=w654:dbl)
      n371 = Multiply(x=1.36603, y=w578) -> (x*y=w593:dbl)
      n372 = Multiply(x=1.36603, y=w714) -> (x*y=w729:dbl)
      n373 = Multiply(x=1.36603, y=w775) -> (x*y=w790:dbl)
      n374 = Multiply(x=w632, y=0.11116) -> (x*y=w631:dbl)
      n375 = Multiply(x=w633, y=-0.47719) -> (x*y=w630:dbl)
      n376 = Multiply(x=w571, y=0.11116) -> (x*y=w570:dbl)
      n377 = Multiply(x=w572, y=-0.47719) -> (x*y=w569:dbl)
      n378 = Multiply(x=w707, y=0.11116) -> (x*y=w706:dbl)
      n379 = Multiply(x=w708, y=-0.47719) -> (x*y=w705:dbl)
      n380 = Multiply(x=w768, y=0.11116) -> (x*y=w767:dbl)
      n381 = Multiply(x=w769, y=-0.47719) -> (x*y=w766:dbl)
      n382 = Compound Arithmetic op=unknown(w631, w630, w654) -> (w606:dbl)
      n383 = Compound Arithmetic op=unknown(w570, w569, w593) -> (w546:dbl)
      n384 = Compound Arithmetic op=unknown(w706, w705, w729) -> (w682:dbl)
      n385 = Compound Arithmetic op=unknown(w767, w766, w790) -> (w742:dbl)
      n386 = Subtract(x=w600, y=w606) -> (x-y=w603:dbl)
      n387 = Multiply(x=w606, y=w608) -> (x*y=w607:dbl)
      n388 = Subtract(x=w540, y=w546) -> (x-y=w543:dbl)
      n389 = Multiply(x=w546, y=w535) -> (x*y=w547:dbl)
      n390 = Subtract(x=w676, y=w682) -> (x-y=w679:dbl)
      n391 = Multiply(x=w682, y=w671) -> (x*y=w683:dbl)
      n392 = Subtract(x=w736, y=w742) -> (x-y=w739:dbl)
      n393 = Multiply(x=w742, y=w744) -> (x*y=w743:dbl)
      n394 = Multiply(x=w612, y=w603) -> (x*y=w604:dbl)
      n395 = Multiply(x=w551, y=w543) -> (x*y=w544:dbl)
      n396 = Multiply(x=w687, y=w679) -> (x*y=w680:dbl)
      n397 = Multiply(x=w748, y=w739) -> (x*y=w740:dbl)
      n398 = Add(x=w604, y=w607) -> (x+y=w599:dbl)
      n399 = Add(x=w544, y=w547) -> (x+y=w539:dbl)
      n400 = Add(x=w680, y=w683) -> (x+y=w675:dbl)
      n401 = Add(x=w740, y=w743) -> (x+y=w735:dbl)
      n402 = Multiply(x=w599, y=w519) -> (x*y=w598:dbl)
      n403 = Multiply(x=w539, y=w519) -> (x*y=w538:dbl)
      n404 = Multiply(x=w675, y=w663) -> (x*y=w674:dbl)
      n405 = Multiply(x=w735, y=w663) -> (x*y=w734:dbl)
      n406 = Subtract(x=w600, y=w598) -> (x-y=w532:dbl)
      n407 = Subtract(x=w540, y=w538) -> (x-y=w531:dbl)
      n408 = Subtract(x=w676, y=w674) -> (x-y=w666:dbl)
      n409 = Subtract(x=w736, y=w734) -> (x-y=w667:dbl)
      n410 = case shown="False" w534 {
        tunnel: [w811 w817] -> w518
        tunnel: w519 -> [_ w818]
        tunnel: w533 -> [w814 _]
        tunnel: w532 -> [w813 _]
        tunnel: w531 -> [w812 _]
        frame False {
          n411 = case shown="False" w814 {
            tunnel: [w815 w816] -> w811
            tunnel: w813 -> [_ w816]
            tunnel: w812 -> [w815 _]
            frame False {
            }
            frame True {
            }
          }
        }
        frame True {
          n412 = Subtract(x=1.0, y=w818) -> (x-y=w817:dbl)
        }
      }
      n413 = case shown="False" w670 {
        tunnel: [w820 w826] -> w669
        tunnel: w663 -> [_ w827]
        tunnel: w668 -> [w823 _]
        tunnel: w667 -> [w822 _]
        tunnel: w666 -> [w821 _]
        frame False {
          n414 = case shown="False" w823 {
            tunnel: [w824 w825] -> w820
            tunnel: w822 -> [_ w825]
            tunnel: w821 -> [w824 _]
            frame False {
            }
            frame True {
            }
          }
        }
        frame True {
          n415 = Subtract(x=1.0, y=w827) -> (x-y=w826:dbl)
        }
      }
      n416 = Multiply(x=w518, y=w500) -> (x*y=w501:dbl)
      n417 = Multiply(x=w669, y=w511) -> (x*y=w510:dbl)
      n418 = case shown="False" w504 {
        tunnel: 0.0 -> [w796 w803]
        tunnel: w511 -> [w795 w810]
        tunnel: w510 -> [w794 w809]
        tunnel: "AFP Efficiency" -> [_ w797]
        tunnel: [w794 w805] -> w508
        tunnel: [w795 w804] -> w507
        tunnel: [w796 w803] -> w506
        tunnel: w501 -> [w793 w802]
        tunnel: [w793 w801] -> w502
        tunnel: w500 -> [w792 w800]
        tunnel: [w792 w798] -> w499
        frame False {
        }
        frame True {
          n419 = Negate(x=w800) -> (-x=w799:dbl)
          n420 = Negate(x=w802) -> (-x=w808:dbl)
          n421 = Negate(x=w809) -> (-x=w807:dbl)
          n422 = Negate(x=w810) -> (-x=w806:dbl)
          n423 = Multiply(x=w799, y=w797) -> (x*y=w798:dbl)
          n424 = Multiply(x=w808, y=w797) -> (x*y=w801:dbl)
          n425 = Multiply(x=w807, y=w797) -> (x*y=w805:dbl)
          n426 = Multiply(x=w806, y=w797) -> (x*y=w804:dbl)
        }
      }
    }
    n427 = Divide(x=12.0, y=500.0) -> (x/y=w105:dbl)
    n428 = Divide(x=12.0, y=500.0) -> (x/y=w143:dbl)
    n429 = Divide(x=12.0, y=500.0) -> (x/y=w147:dbl)
    n430 = Divide(x=12.0, y=500.0) -> (x/y=w101:dbl)
    n431 = Multiply(x=w97, y=w105) -> (x*y=→"upper R-value AFP":dbl)
    n432 = Multiply(x=w136, y=w143) -> (x*y=→"lower R-value":dbl)
    n433 = Multiply(x=w139, y=w147) -> (x*y=→"upper R-value":dbl)
    n434 = Multiply(x=w94, y=w101) -> (x*y=→"lower R-value AFP":dbl)
    n435 = case shown="True" w185 {
      tunnel: w189 -> [_ w488]
      tunnel: w88 -> [w484 w487]
      tunnel: w88 -> [_ w486]
      tunnel: [w484 w486] -> w188
      tunnel: [w483 w485] -> w176
      tunnel: w179 -> [w483 _]
      frame False {
      }
      frame True {
        n436 = Subtract(x=w488, y=w487) -> (x-y=w485:dbl[])
      }
    }
    n437 = case shown="True" w185 {
      tunnel: w203 -> [_ w494]
      tunnel: w194 -> [w490 w493]
      tunnel: w202 -> [_ w492]
      tunnel: [w490 w492] -> w186
      tunnel: [w489 w491] -> w175
      tunnel: w179 -> [w489 _]
      frame False {
      }
      frame True {
        n438 = Subtract(x=w494, y=w493) -> (x-y=w491:dbl[])
      }
    }
    n439 = Add(x=w188, y=w78) -> (x+y=w68:dbl[])
    n440 = Add(x=w176, y=w78) -> (x+y=w70:dbl[])
    n441 = Add(x=w79, y=w175) -> (x+y=w72:dbl[])
    n442 = Add(x=w79, y=w186) -> (x+y=w74:dbl[])
    n443 = call "FitAndSubtract.vi"("Array 4"=w65, "Array 3"=w66, "Numeric"=w67, "Array in"=w68) -> ("Array out"=w69:dbl[])  [unwired: 6 in, 1 out]
    n444 = call "FitAndSubtract.vi"("Array 4"=w65, "Array 3"=w66, "Numeric"=w67, "Array in"=w70) -> ("Array out"=w71:dbl[])  [unwired: 6 in, 1 out]
    n445 = call "FitAndSubtract.vi"("Array 4"=w65, "Array 3"=w66, "Numeric"=w67, "Array in"=w72) -> ("Array out"=w75:dbl[])  [unwired: 6 in, 1 out]
    n446 = Bundle(w66, w74) -> (w228:cluster{dbl[], dbl[]})  [unwired: 1 in]
    n447 = call "FitAndSubtract.vi"("Array 4"=w65, "Array 3"=w66, "Numeric"=w67, "Array in"=w74) -> ("Best Polynomial Fit"=w73:dbl[], "Array out"=w76:dbl[])  [unwired: 6 in]
    n448 = Bundle(w66, "Best Polynomial Fit"=w73) -> (w162:cluster{dbl[], "Best Polynomial Fit":dbl[]})  [unwired: 1 in]
    n449 = call "rhozero.vi"("Array in"=w69) -> ("Array out"=w183:dbl[])  [unwired: 10 in]
    n450 = call "rhominus.vi"("Array"=w76, "Array 2"=w69) -> ("Array 3"=w182:dbl[])  [unwired: 9 in]
    n451 = Add(x=w75, y=w71) -> (x+y=w177:dbl[])
    n452 = Subtract(x=w75, y=w71) -> (x-y=w178:dbl[])
    n453 = call "rhoplus.vi"("Array 3"=w69, "Array in"=w76) -> ("Array out"=w184:dbl[])  [unwired: 9 in]
    n454 = Build Array(w228, w162) -> (→"Signal and Fit (P)":cluster{dbl[], "Best Polynomial Fit":dbl[]}[])
    n455 = Divide(x=w177, y=w174) -> (x/y=w173:dbl[])
    n456 = Subtract(x=w184, y=w183) -> (x-y=w171:dbl[])
    n457 = Divide(x=w178, y=w174) -> (x/y=w172:dbl[])
    n458 = Bundle(w66, "Array out"=w183) -> (→"Rho_0":cluster{dbl[], "Array out":dbl[]})  [unwired: 1 in]
    n459 = Bundle(w66, "Array out"=w184) -> (→"Rho_+":cluster{dbl[], "Array out":dbl[]})  [unwired: 1 in]
    n460 = Subtract(x=w183, y=w182) -> (x-y=w170:dbl[])
    n461 = Bundle(w66, "Array 3"=w182) -> (→"Rho_-":cluster{dbl[], "Array 3":dbl[]})  [unwired: 1 in]
    n462 = Reverse 1D Array(array=w173) -> (reversed array=w181:dbl[])
    n463 = Reverse 1D Array(array=w172) -> (reversed array=w180:dbl[])
    n464 = Divide(x=w181, y=w174) -> (x/y=w82:dbl[])
    n465 = Divide(x=w180, y=w174) -> (x/y=w83:dbl[])
    n466 = Add(x=w170, y=w82) -> (x+y=w168:dbl[])
    n467 = Add(x=w171, y=w83) -> (x+y=w169:dbl[])
    n468 = Subtract(x=w169, y=w168) -> (x-y=w156:dbl[])
    n469 = Add(x=w168, y=w169) -> (x+y=w60:dbl[])
    n470 = Bundle(w66, w169) -> (w163:cluster{dbl[], dbl[]})  [unwired: 1 in]
    n471 = Bundle(w66, w168) -> (w164:cluster{dbl[], dbl[]})  [unwired: 1 in]
    n472 = Add Array Elements(numeric array=w60) -> (sum=w158:dbl)
    n473 = Add Array Elements(numeric array=w156) -> (sum=w157:dbl)
    n474 = Bundle(w66, w156) -> (→"Corrected Data (Q)":cluster{dbl[], dbl[]})  [unwired: 1 in]
    n475 = Bundle(w66, w60) -> (w165:cluster{dbl[], dbl[]})  [unwired: 1 in]
    n476 = Array To Spreadsheet String(delimiter (Tab)=",", array=w60, 3:"%f") -> (spreadsheet string=w64:string)
    n477 = Format Into String(format string="%d", initial string="", w53) -> (resulting string=w118:string)  [unwired: 1 in, 1 out]
    n478 = Build Array(w165, w163, w164) -> (→"Corrected Data (P)":cluster{dbl[], dbl[]}[])
    n479 = Number To Fractional String(number="Saturation\nPolarization", precision (6)=i16 2) -> (F-format string=w62:string)  [unwired: 2 in]
    n480 = Divide(x=12.0, y=500.0) -> (x/y=w154:dbl)
    n481 = Divide(x=12.0, y=500.0) -> (x/y=w148:dbl)
    n482 = Multiply(x=w158, y=w154) -> (x*y=w155:dbl)
    n483 = Multiply(x=w157, y=w148) -> (x*y=w151:dbl)
    n484 = Absolute Value(x=w155) -> (abs(x)=w108:dbl)
    "Reimann\nsum of P" <- w108
    n485 = Concatenate Strings(w118, ",", w62, ",", w64) -> (w115:string)
    n486 = Absolute Value(x=w151) -> (abs(x)=w135:dbl)
    "Reimann \nsum of Q" <- w135
    n487 = Write to Text File(file (use dialog)=w124, text=w115, error in=w123) -> (refnum out=w122:refnum<file>, error out=w121:errorcluster)  [unwired: 1 in, 1 out]
    n488 = Square(x=w108) -> (x^2=w106:dbl)
    n489 = Bundle(w108, w135) -> (→"Total Polarization (P)":cluster{dbl, dbl})  [unwired: 1 in]
    n490 = Quotient & Remainder(x=w53, y="Batch Size") -> (x-y*floor(x/y)=w51:i32)  [unwired: 1 out]
    n491 = Multiply(x=3, y=w106) -> (x*y=w110:dbl)
    n492 = Equal To 0?(x=w51) -> (x = 0?=w50:bool)
    n493 = Select(t="Training?", s=w50, f=FALSE) -> (s? t:f=w47:bool)
    n494 = call "Ann_int.vi"("Data"=w60, "Loss Function"="Loss Function", "Regularization"="Regularization", "Target"="Saturation\nPolarization", "Training?"=w47, "Parameters"=w58, "Adam Data In"=w54) -> ("Output"=→"NN Output":dbl, "Error"=w44:dbl, "Adjusted Parameters"=w42:T4, "Adam Data Out"=w55:T2)  [unwired: 5 in]
    "NN Error" <- w44
    "NN Loss" <- w44
    n495 = Subtract(x=4, y=w110) -> (x-y=w107:dbl)
    n496 = Square Root(x=w107) -> (sqrt(x)=w112:dbl)
    n497 = Less?(x=w45, y=w44) -> (x < y?=w43:bool)
    n498 = Subtract(x=2, y=w112) -> ()  [unwired: 1 out]
    n499 = Select(t=w45, s=w43, f=w44) -> (s? t:f=w46:dbl)
    n500 = Select(t=w40, s=w43, f=w42) -> (s? t:f=w41:T4)
  }
  n501 = invoke class="VI" method="Default Vals.Reinit All"(reference=w38) -> ()  [unwired: 2 in, 3 out]
  n502 = property on="Total Polarization (P)" class="WFChart (strict)"("History Data"=cluster{dbl, dbl}[] []) -> ()  [unwired: 2 in, 2 out]
  n503 = property on="NN Training Loss" class="WFChart (strict)"("History Data"=dbl[] []) -> ()  [unwired: 2 in, 2 out]
  n504 = Close File(refnum=w34, error in=w33) -> ()  [unwired: 2 out]
  n505 = Flatten To XML(anything=w2) -> (xml string=w30:string)
  n506 = call-poly <vilib>:"Write to XML File.vi"("XML Input"=w30, "XML File Path"="Parameters File Path") -> ()  [unwired: 7 in, 3 out]
